vi "Set Experiment Start Datetime.vi"(8 "error in (no error)":errorcluster, 9 "start datetime":timestamp, 10 "experiment id":u32, 11 "eLab in":refnum<class "PL eLabFTW Client.lvclass">) -> (0 "error out":errorcluster, 3 "eLab out":refnum<class "PL eLabFTW Client.lvclass">)   [LabVIEW 2015, in "PL eLabFTW Client.lvclass"]
doc: "Sets experiment start datetime."
uses:
  PL eLabFTW Client.lvclass
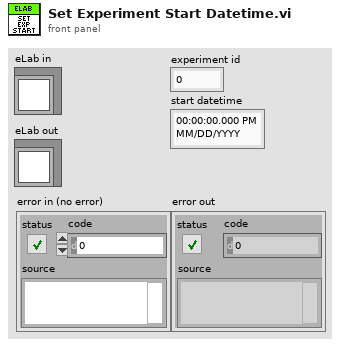
[diagram p1: front panel]
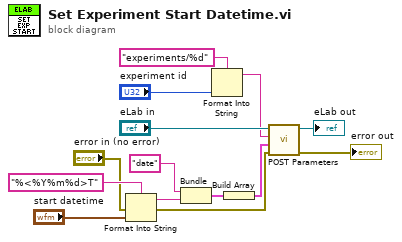
[diagram p0: block diagram]
diagram:
  n1 = Format Into String(format string="%<%Y%m%d>T", error in="error in (no error)", "start datetime") -> (resulting string=w5:string, error out=w2:errorcluster)  [unwired: 1 in]
  n2 = Bundle("format string"="date", w5) -> (w7:cluster{"format string":string, string})  [unwired: 1 in]
  n3 = Format Into String(format string="experiments/%d", "experiment id") -> (resulting string=w9:string)  [unwired: 2 in, 1 out]
  n4 = Build Array(w7) -> (w1:cluster{"format string":string, string}[])
  n5 = call "POST Parameters.vi"("error in (no error)"=w2, "parameters"=w1, "relative URL"=w9, "eLab in"="eLab in") -> ("error out"=→"error out":errorcluster, "eLab out"=→"eLab out":refnum<class "PL eLabFTW Client.lvclass">)  [unwired: 5 in, 1 out]
